vi "USBClient1Sub.vi"() -> ()   [LabVIEW 2018]
uses:
  <vilib>/daq.io/MQTT LabVIEW Client/Controls/Connect_Flags.ctl
  <vilib>/daq.io/MQTT LabVIEW Client/Controls/QoS.ctl
  <vilib>/daq.io/MQTT LabVIEW Client/Controls/DUP_Flag.ctl
  <vilib>/daq.io/MQTT LabVIEW Client/Controls/Retain_Flag.ctl
  <vilib>/DAQmx/write.llb/DAQmx Write (Digital Bool 1Line 1Point).vi
  <vilib>/DAQmx/create/channels.llb/DAQmx Create Channel (DO-Digital Output).vi
  <vilib>/DAQmx/miscellaneous.llb/DAQmx Fill In Error Info.vi
  <vilib>/daq.io/MQTT LabVIEW Client/MQTT_Functions.lvlib
panel:
  in  "stop":bool
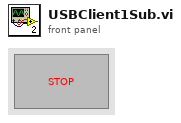
[diagram p1: front panel]
types:
  T1 = typedef "MQTT_Functions.lvlib/QoS.ctl" = enum8{"At most once", "At least once", "Exactly once", "Reserved"}
  T2 = typedef "MQTT_Functions.lvlib/DUP_Flag.ctl" = bool
  T3 = typedef "MQTT_Functions.lvlib/Retain_Flag.ctl" = bool
  T4 = cluster{"QoS":T1, "DUP":T2, "Retain":T3, "Keep Alive (sec)":u16}
  T5 = typedef "MQTT_Functions.lvlib/Connect_Flags.ctl" = cluster{"user name":bool, "password":bool, "will retain":bool, "will flag":bool, "clean session":bool, "reserved":bool, "will QoS":T1}
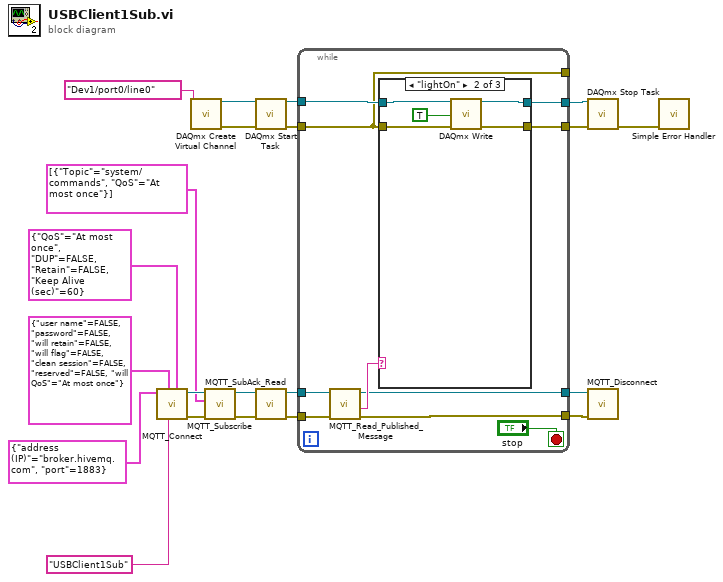
[diagram p0: block diagram]
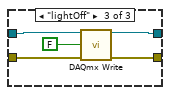
[diagram p3: hidden frame]
diagram:
  n1 = call <vilib>:"MQTT_Connect.vi"("Connect Meta"=T4 {"QoS"=enum."At most once", "DUP"=FALSE, "Retain"=FALSE, "Keep Alive (sec)"=60}, "Client ID"="USBClient1Sub", "Connect Flags"=T5 {"user name"=FALSE, "password"=FALSE, "will retain"=FALSE, "will flag"=FALSE, "clean session"=FALSE, "reserved"=FALSE, "will QoS"=enum."At most once"}, "MQTT Broker"=cluster{"address (IP)":string, "port":u16} {"address (IP)"="broker.hivemq.com", "port"=1883}) -> ("error out"=w17:errorcluster, "connection ID out"=w16:refnum<k5>)  [unwired: 5 in, 1 out]
  n2 = call-poly <vilib>:"DAQmx Create Virtual Channel.vi"("lines"=tag "Dev1/port0/line0") -> ("task out"=w10:refnum<k21>, "error out"=w9:errorcluster)  [unwired: 13 in]
  n3 = call <vilib>:"MQTT_Subscribe.vi"("error in (no error)"=w17, "Subscription Info Array"=cluster{"Topic":string, "QoS":T1}[] [{"Topic"="system/commands", "QoS"=enum."At most once"}], "connection ID"=w16) -> ("error out"=w14:errorcluster, "connection ID out"=w13:refnum<k5>)  [unwired: 7 in]
  n4 = call <vilib>:"DAQmx Start Task.vi"("task/channels in"=w10, "error in"=w9) -> ("task out"=w8:refnum<k21>, "error out"=w7:errorcluster)  [unwired: 12 in]
  n5 = call <vilib>:"MQTT_SubAck_Read.vi"("error in (no error)"=w14, "connection ID"=w13) -> ("error out"=w11:errorcluster, "connection ID out"=w12:refnum<k5>)  [unwired: 7 in, 1 out]
  n6 = while {
    tunnel: w12 -> [w31]
    tunnel: w11 -> [w30]
    tunnel: w8 -> [w27]
    tunnel: [w26] -> _
    tunnel: w7 -> [w26]
    tunnel: [w28] -> w4
    tunnel: [w25] -> w6
    tunnel: [w24] -> w5
    tunnel: [w22] -> w3
    stop <- "stop" stop-if-true
    n7 = call <vilib>:"MQTT_Read_Published_Message.vi"("error in (no error)"=w30, "connection ID"=w31) -> ("error out"=w22:errorcluster, "Message"=w29:string, "connection ID out"=w28:refnum<k5>)  [unwired: 4 in, 3 out]
    n8 = case shown="\"lightOn\"" w29 {
      tunnel: w27 -> [w33 w38 w43]
      tunnel: w26 -> [w32 w37 w42]
      tunnel: [w33 w36 w41] -> w25
      tunnel: [w32 w35 w40] -> w24
      frame "false", Default {
      }
      frame "lightOn" {
        n9 = call-poly <vilib>:"DAQmx Write.vi"("task/channels in"=w38, "data"=TRUE, "error in"=w37) -> ("task out"=w36:refnum<k21>, "error out"=w35:errorcluster)  [unwired: 10 in, 1 out]
      }
      frame "lightOff" {
        n10 = call-poly <vilib>:"DAQmx Write.vi"("task/channels in"=w43, "data"=FALSE, "error in"=w42) -> ("task out"=w41:refnum<k21>, "error out"=w40:errorcluster)  [unwired: 10 in, 1 out]
      }
    }
  }
  n11 = call <vilib>:"DAQmx Stop Task.vi"("task/channels in"=w6, "error in"=w5) -> ("error out"=w2:errorcluster)  [unwired: 12 in, 1 out]
  n12 = call <vilib>:"MQTT_Disconnect.vi"("error in (no error)"=w3, "connection ID"=w4) -> ()  [unwired: 9 in, 1 out]
  n13 = call <vilib>:"Simple Error Handler.vi"("error in (no error)"=w2) -> ()  [unwired: 4 in, 5 out]
